vi "test pulse.vi"() -> ()   [LabVIEW 2012]
uses:
  <vilib>/DAQmx/read.llb/DAQmx Read (Digital Bool 1Line 1Point).vi
  <vilib>/DAQmx/create/channels.llb/DAQmx Create Channel (DI-Digital Input).vi
  <vilib>/DAQmx/miscellaneous.llb/DAQmx Fill In Error Info.vi
  <vilib>/express/express arith-compare/Formula/XNode/ExpressFormulaBlockNode.xnode
panel:
  in  "Pi Pulse":bool
  in  "MW post pause":dbl
  in  "Rabi Freq":dbl
  out "Array":dbl[](array[numeric])
  in  "AOM pause + MW delay":dbl
  in  "Sweep range":dbl
  in  "Step size":dbl
  in  "N Loop":i32=25000
  in  "APD signal width":dbl
  out "Run":bool
  in  "AOM Pulse length":dbl=3e-07
  in  "Path to spinapi.dll":path=path "C:/SpinCore/SpinAPI/dll/spinapi64.dll"
  in  "stop":bool
  in  "start/restart":bool
  in  "clock_freq (MHz)":dbl=300.0
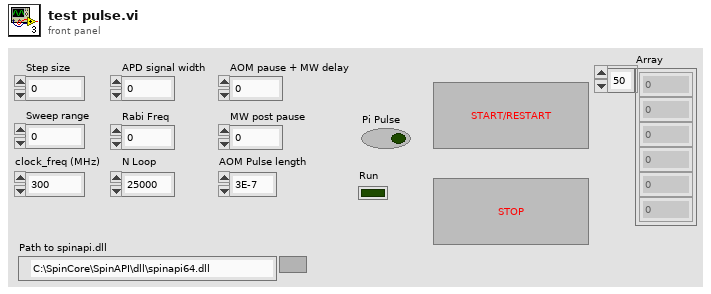
[diagram p1: front panel]
types:
  T1 = cluster{"Instruct Data":i32, "Op Code":i32, "Flags":bool[], "Comments":string, "Time (s)":dbl}[]
  T2 = cluster{"Instruct Data":i32, "Op Code":i32, "Flags":bool[], "Comments":string, "Time (s)":dbl}
  T3 = enum16{"Pulse Program", "Frequency Registers", "TX Phase Registers", "RX Phase Registers"}
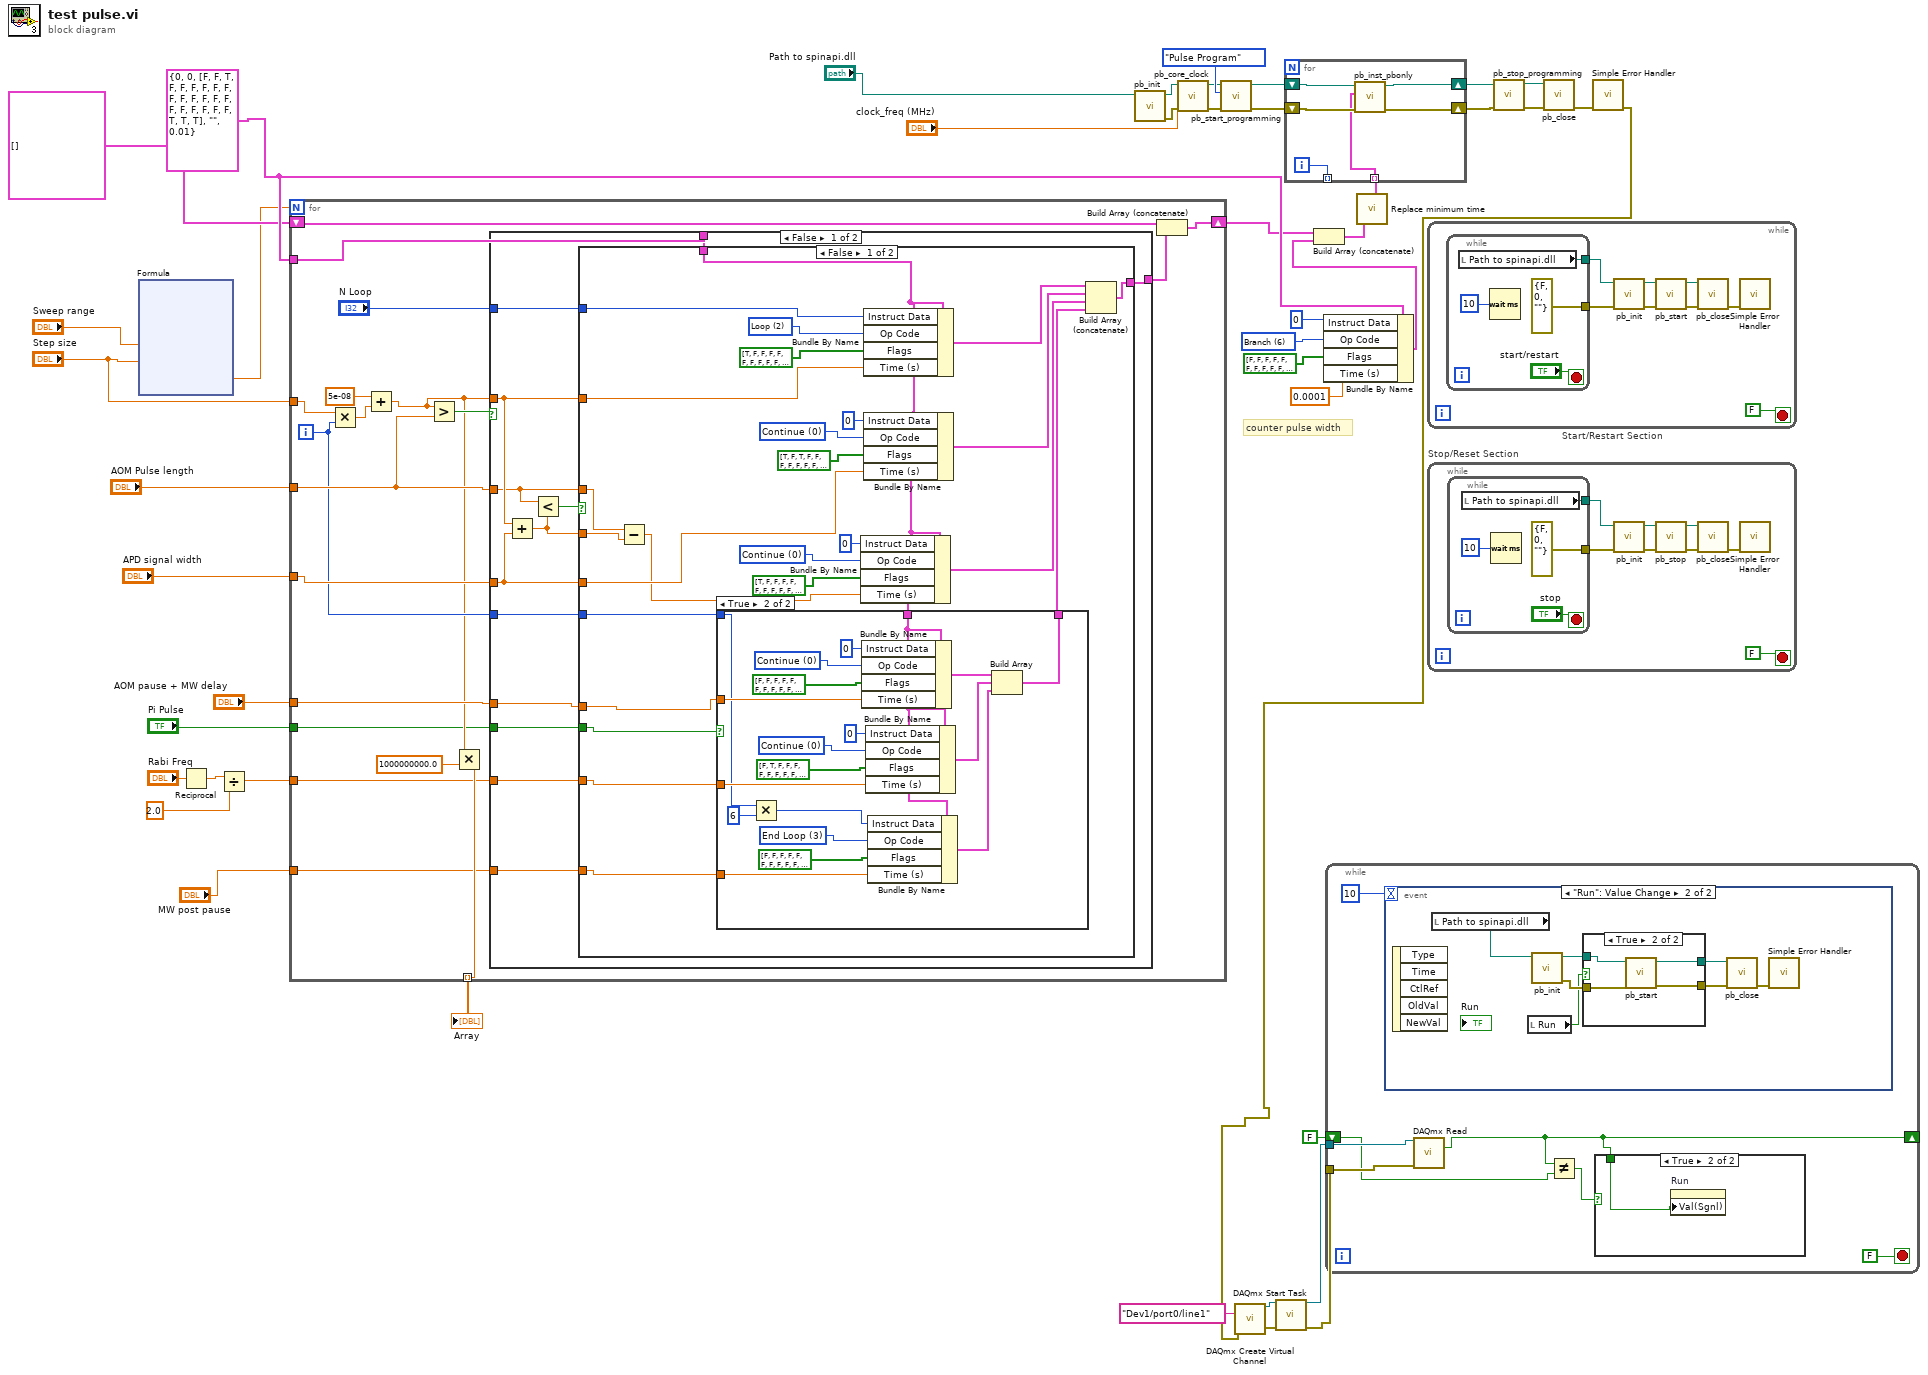
[diagram p0: block diagram]
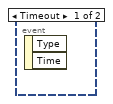
[diagram p2: hidden frame]
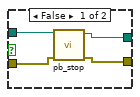
[diagram p3: hidden frame]
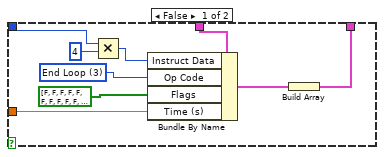
[diagram p5: hidden frame]
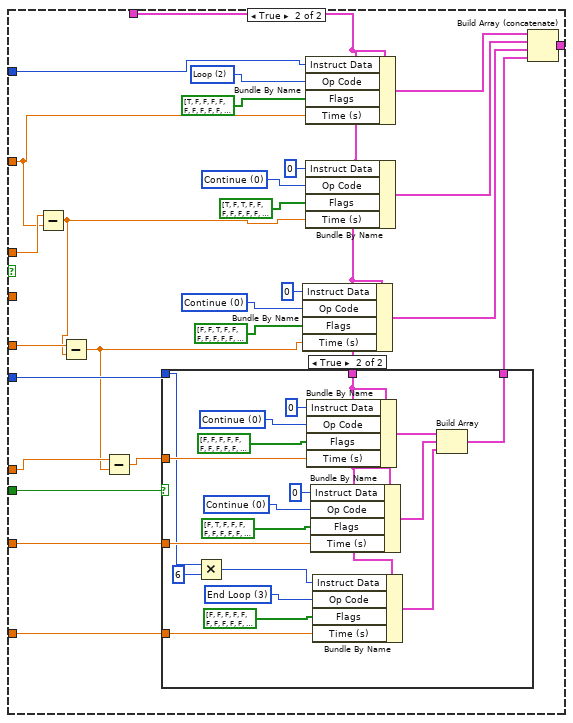
[diagram p6: hidden frame]
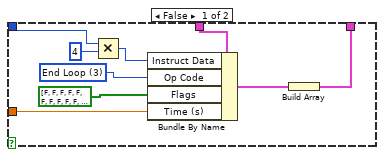
[diagram p7: hidden frame]
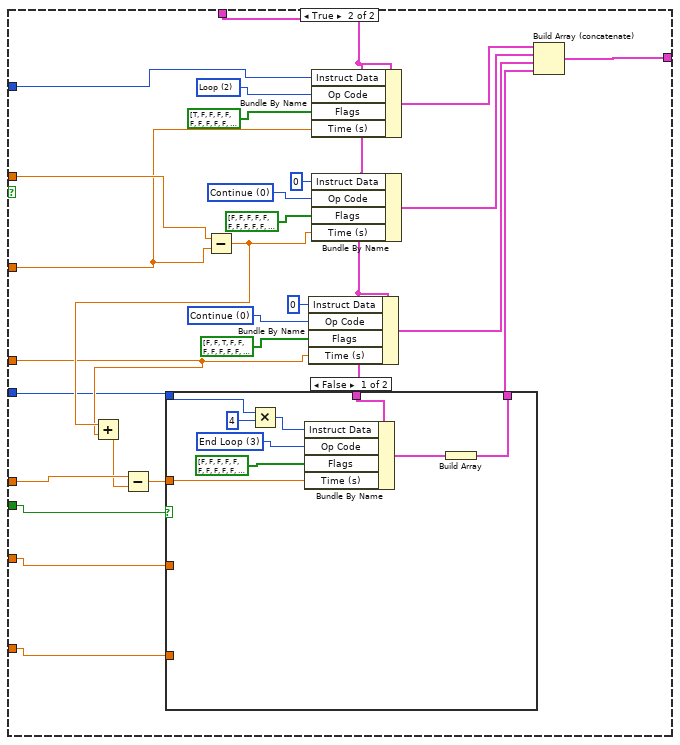
[diagram p8: hidden frame]
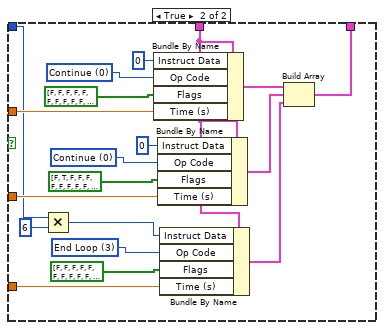
[diagram p9: hidden frame]
diagram:
  w21 = 6 items=["Continue", "Stop", "Loop", "End Loop", "JSR", "RTS", "Branch", "Long Delay", "Wait"] ("Op Code")
  w19 = T2 {"Instruct Data"=0, "Op Code"=0, "Flags"=[FALSE, FALSE, TRUE, FALSE, FALSE, FALSE, FALSE, FALSE, FALSE, FALSE, FALSE, FALSE, FALSE, FALSE, FALSE, FALSE, FALSE, FALSE, FALSE, FALSE, FALSE, TRUE, TRUE, TRUE], "Comments"="", "Time (s)"=0.01} ("PB Inst 2")
  # "counter pulse width"
  n1 = xnode "Formula"("X1"="Sweep range", "X2"="Step size") -> ("Result"=w1:dbl)  [unwired: 1 in, 1 out]
  n2 = Reciprocal(x="Rabi Freq") -> (1/x=w8:dbl)
  n3 = Divide(x=w8, y=2.0) -> (x/y=w7:dbl)
  n4 = for {
    N: w1 -> [_]
    tunnel: w19 -> [w60]
    shift-right: [w62] -> w17
    shift-left: T1 [] -> [w63]
    tunnel: "AOM Pulse length" -> [w54]
    tunnel: "Step size" -> [w58]
    tunnel: "APD signal width" -> [w53]
    tunnel: "AOM pause + MW delay" -> [w51]
    tunnel: [w49] -> w10 mode=indexing
    tunnel: w7 -> [w47]
    tunnel: "MW post pause" -> [w46]
    tunnel: "Pi Pulse" -> [w45]
    i -> [w52]
    n5 = Multiply(x=w58, y=w52) -> (x*y=w57:dbl)
    n6 = Add(x=5e-08, y=w57) -> (x+y=w50:dbl)
    n7 = Greater?(x=w50, y=w54) -> (0:w55:bool)
    n8 = Multiply(x=w50, y=1000000000.0) -> (x*y=w49:dbl)
    n9 = case shown="False" w55 {
      tunnel: [w75 w203] -> w61
      tunnel: w60 -> [w76 w185]
      tunnel: "N Loop" -> [w67 w202]
      tunnel: w54 -> [w72 w195]
      tunnel: w50 -> [w73 w196]
      tunnel: w53 -> [w71 w193]
      tunnel: w52 -> [w70 w190]
      tunnel: w51 -> [w69 w192]
      tunnel: w47 -> [w66 w187]
      tunnel: w46 -> [w65 w186]
      tunnel: w45 -> [w64 w188]
      frame False {
        n10 = Add(x=w73, y=w71) -> (x+y=w68:dbl)
        n11 = Less?(x=w72, y=w68) -> (x < y?=w74:bool)
        n12 = case shown="False" w74 {
          tunnel: w76 -> [w78 w144]
          tunnel: [w90 w142] -> w75
          tunnel: w73 -> [w89 w140]
          tunnel: w72 -> [w87 w141]
          tunnel: w71 -> [w88 w139]
          tunnel: w70 -> [w83 w137]
          tunnel: w69 -> [w82 w136]
          tunnel: w68 -> [w86 _]
          tunnel: w67 -> [w84 w133]
          tunnel: w66 -> [w80 w132]
          tunnel: w65 -> [w79 w131]
          tunnel: w64 -> [w81 w130]
          frame False {
            w99 = 0 items=["Continue", "Stop", "Loop", "End Loop", "JSR", "RTS", "Branch", "Long Delay", "Wait"] ("Op Code")
            w96 = 2 items=["Continue", "Stop", "Loop", "End Loop", "JSR", "RTS", "Branch", "Long Delay", "Wait"] ("Op Code")
            w92 = 0 items=["Continue", "Stop", "Loop", "End Loop", "JSR", "RTS", "Branch", "Long Delay", "Wait"] ("Op Code")
            n13 = Subtract(x=w87, y=w86) -> (x-y=w85:dbl)
            n14 = case shown="True" w81 {
              tunnel: [w102 w111] -> w77
              tunnel: w78 -> [w107 w119]
              tunnel: w83 -> [w106 w117]
              tunnel: w82 -> [w105 w126]
              tunnel: w80 -> [_ w122]
              tunnel: w79 -> [_ w118]
              frame False {
                w104 = 3 items=["Continue", "Stop", "Loop", "End Loop", "JSR", "RTS", "Branch", "Long Delay", "Wait"] ("Op Code")
                n15 = Multiply(x=w106, y=4) -> (x*y=w109:i32)
                n16 = Bundle By Name(cluster=w107, "Instruct Data"=w109, "Op Code"=w104, "Flags"=bool[] [FALSE, FALSE, FALSE, FALSE, FALSE, FALSE, FALSE, FALSE, FALSE, FALSE, FALSE, FALSE, FALSE, FALSE, FALSE, FALSE, FALSE, FALSE, FALSE, FALSE, FALSE, TRUE, TRUE, TRUE], "Time (s)"=w105) -> (w103:T2)
                n17 = Build Array(w103) -> (w102:T1)
              }
              frame True {
                w121 = 3 items=["Continue", "Stop", "Loop", "End Loop", "JSR", "RTS", "Branch", "Long Delay", "Wait"] ("Op Code")
                w125 = 0 items=["Continue", "Stop", "Loop", "End Loop", "JSR", "RTS", "Branch", "Long Delay", "Wait"] ("Op Code")
                w129 = 0 items=["Continue", "Stop", "Loop", "End Loop", "JSR", "RTS", "Branch", "Long Delay", "Wait"] ("Op Code")
                n18 = Multiply(x=w117, y=6) -> (x*y=w115:i32)
                n19 = Bundle By Name(cluster=w119, "Instruct Data"=0, "Op Code"=w129, "Flags"=bool[] [FALSE, FALSE, FALSE, FALSE, FALSE, FALSE, FALSE, FALSE, FALSE, FALSE, FALSE, FALSE, FALSE, FALSE, FALSE, FALSE, FALSE, FALSE, FALSE, FALSE, FALSE, TRUE, TRUE, TRUE], "Time (s)"=w126) -> (w112:T2)
                n20 = Bundle By Name(cluster=w119, "Instruct Data"=0, "Op Code"=w125, "Flags"=bool[] [FALSE, TRUE, FALSE, FALSE, FALSE, FALSE, FALSE, FALSE, FALSE, FALSE, FALSE, FALSE, FALSE, FALSE, FALSE, FALSE, FALSE, FALSE, FALSE, FALSE, FALSE, TRUE, TRUE, TRUE], "Time (s)"=w122) -> (w113:T2)
                n21 = Bundle By Name(cluster=w119, "Instruct Data"=w115, "Op Code"=w121, "Flags"=bool[] [FALSE, FALSE, FALSE, FALSE, FALSE, FALSE, FALSE, FALSE, FALSE, FALSE, FALSE, FALSE, FALSE, FALSE, FALSE, FALSE, FALSE, FALSE, FALSE, FALSE, FALSE, TRUE, TRUE, TRUE], "Time (s)"=w118) -> (w114:T2)
                n22 = Build Array(w112, w113, w114) -> (w111:T1)
              }
            }
            n23 = Bundle By Name(cluster=w78, "Instruct Data"=0, "Op Code"=w92, "Flags"=bool[] [TRUE, FALSE, FALSE, FALSE, FALSE, FALSE, FALSE, FALSE, FALSE, FALSE, FALSE, FALSE, FALSE, FALSE, FALSE, FALSE, FALSE, FALSE, FALSE, FALSE, FALSE, TRUE, TRUE, TRUE], "Time (s)"=w85) -> (w95:T2)
            n24 = Bundle By Name(cluster=w78, "Instruct Data"=w84, "Op Code"=w96, "Flags"=bool[] [TRUE, FALSE, FALSE, FALSE, FALSE, FALSE, FALSE, FALSE, FALSE, FALSE, FALSE, FALSE, FALSE, FALSE, FALSE, FALSE, FALSE, FALSE, FALSE, FALSE, FALSE, TRUE, TRUE, TRUE], "Time (s)"=w89) -> (w101:T2)
            n25 = Bundle By Name(cluster=w78, "Instruct Data"=0, "Op Code"=w99, "Flags"=bool[] [TRUE, FALSE, TRUE, FALSE, FALSE, FALSE, FALSE, FALSE, FALSE, FALSE, FALSE, FALSE, FALSE, FALSE, FALSE, FALSE, FALSE, FALSE, FALSE, FALSE, FALSE, TRUE, TRUE, TRUE], "Time (s)"=w88) -> (w94:T2)
            n26 = Build Array (concatenate)(w101, w94, w95, w77) -> (w90:T1)
          }
          frame True {
            w146 = 0 items=["Continue", "Stop", "Loop", "End Loop", "JSR", "RTS", "Branch", "Long Delay", "Wait"] ("Op Code")
            w149 = 2 items=["Continue", "Stop", "Loop", "End Loop", "JSR", "RTS", "Branch", "Long Delay", "Wait"] ("Op Code")
            w154 = 0 items=["Continue", "Stop", "Loop", "End Loop", "JSR", "RTS", "Branch", "Long Delay", "Wait"] ("Op Code")
            n27 = Subtract(x=w141, y=w140) -> (x-y=w138:dbl)
            n28 = Subtract(x=w139, y=w138) -> (x-y=w135:dbl)
            n29 = Subtract(x=w136, y=w135) -> (x-y=w134:dbl)
            n30 = case shown="True" w130 {
              tunnel: [w156 w165] -> w150
              tunnel: w144 -> [w161 w173]
              tunnel: w137 -> [w160 w171]
              tunnel: w134 -> [w159 w180]
              tunnel: w132 -> [_ w176]
              tunnel: w131 -> [_ w172]
              frame False {
                w158 = 3 items=["Continue", "Stop", "Loop", "End Loop", "JSR", "RTS", "Branch", "Long Delay", "Wait"] ("Op Code")
                n31 = Multiply(x=w160, y=4) -> (x*y=w163:i32)
                n32 = Bundle By Name(cluster=w161, "Instruct Data"=w163, "Op Code"=w158, "Flags"=bool[] [FALSE, FALSE, FALSE, FALSE, FALSE, FALSE, FALSE, FALSE, FALSE, FALSE, FALSE, FALSE, FALSE, FALSE, FALSE, FALSE, FALSE, FALSE, FALSE, FALSE, FALSE, TRUE, TRUE, TRUE], "Time (s)"=w159) -> (w157:T2)
                n33 = Build Array(w157) -> (w156:T1)
              }
              frame True {
                w175 = 3 items=["Continue", "Stop", "Loop", "End Loop", "JSR", "RTS", "Branch", "Long Delay", "Wait"] ("Op Code")
                w179 = 0 items=["Continue", "Stop", "Loop", "End Loop", "JSR", "RTS", "Branch", "Long Delay", "Wait"] ("Op Code")
                w183 = 0 items=["Continue", "Stop", "Loop", "End Loop", "JSR", "RTS", "Branch", "Long Delay", "Wait"] ("Op Code")
                n34 = Multiply(x=w171, y=6) -> (x*y=w169:i32)
                n35 = Bundle By Name(cluster=w173, "Instruct Data"=0, "Op Code"=w183, "Flags"=bool[] [FALSE, FALSE, FALSE, FALSE, FALSE, FALSE, FALSE, FALSE, FALSE, FALSE, FALSE, FALSE, FALSE, FALSE, FALSE, FALSE, FALSE, FALSE, FALSE, FALSE, FALSE, TRUE, TRUE, TRUE], "Time (s)"=w180) -> (w166:T2)
                n36 = Bundle By Name(cluster=w173, "Instruct Data"=0, "Op Code"=w179, "Flags"=bool[] [FALSE, TRUE, FALSE, FALSE, FALSE, FALSE, FALSE, FALSE, FALSE, FALSE, FALSE, FALSE, FALSE, FALSE, FALSE, FALSE, FALSE, FALSE, FALSE, FALSE, FALSE, TRUE, TRUE, TRUE], "Time (s)"=w176) -> (w167:T2)
                n37 = Bundle By Name(cluster=w173, "Instruct Data"=w169, "Op Code"=w175, "Flags"=bool[] [FALSE, FALSE, FALSE, FALSE, FALSE, FALSE, FALSE, FALSE, FALSE, FALSE, FALSE, FALSE, FALSE, FALSE, FALSE, FALSE, FALSE, FALSE, FALSE, FALSE, FALSE, TRUE, TRUE, TRUE], "Time (s)"=w172) -> (w168:T2)
                n38 = Build Array(w166, w167, w168) -> (w165:T1)
              }
            }
            n39 = Bundle By Name(cluster=w144, "Instruct Data"=0, "Op Code"=w154, "Flags"=bool[] [FALSE, FALSE, TRUE, FALSE, FALSE, FALSE, FALSE, FALSE, FALSE, FALSE, FALSE, FALSE, FALSE, FALSE, FALSE, FALSE, FALSE, FALSE, FALSE, FALSE, FALSE, TRUE, TRUE, TRUE], "Time (s)"=w135) -> (w151:T2)
            n40 = Bundle By Name(cluster=w144, "Instruct Data"=w133, "Op Code"=w149, "Flags"=bool[] [TRUE, FALSE, FALSE, FALSE, FALSE, FALSE, FALSE, FALSE, FALSE, FALSE, FALSE, FALSE, FALSE, FALSE, FALSE, FALSE, FALSE, FALSE, FALSE, FALSE, FALSE, TRUE, TRUE, TRUE], "Time (s)"=w140) -> (w143:T2)
            n41 = Bundle By Name(cluster=w144, "Instruct Data"=0, "Op Code"=w146, "Flags"=bool[] [TRUE, FALSE, TRUE, FALSE, FALSE, FALSE, FALSE, FALSE, FALSE, FALSE, FALSE, FALSE, FALSE, FALSE, FALSE, FALSE, FALSE, FALSE, FALSE, FALSE, FALSE, TRUE, TRUE, TRUE], "Time (s)"=w138) -> (w152:T2)
            n42 = Build Array (concatenate)(w143, w152, w151, w150) -> (w142:T1)
          }
        }
      }
      frame True {
        w198 = 0 items=["Continue", "Stop", "Loop", "End Loop", "JSR", "RTS", "Branch", "Long Delay", "Wait"] ("Op Code")
        w201 = 2 items=["Continue", "Stop", "Loop", "End Loop", "JSR", "RTS", "Branch", "Long Delay", "Wait"] ("Op Code")
        w208 = 0 items=["Continue", "Stop", "Loop", "End Loop", "JSR", "RTS", "Branch", "Long Delay", "Wait"] ("Op Code")
        n43 = Subtract(x=w196, y=w195) -> (x-y=w194:dbl)
        n44 = Add(x=w194, y=w193) -> (x+y=w191:dbl)
        n45 = Subtract(x=w192, y=w191) -> (x-y=w189:dbl)
        n46 = case shown="False" w188 {
          tunnel: [w210 w219] -> w184
          tunnel: w185 -> [w215 w227]
          tunnel: w190 -> [w214 w225]
          tunnel: w189 -> [w213 w234]
          tunnel: w187 -> [_ w230]
          tunnel: w186 -> [_ w226]
          frame False {
            w212 = 3 items=["Continue", "Stop", "Loop", "End Loop", "JSR", "RTS", "Branch", "Long Delay", "Wait"] ("Op Code")
            n47 = Multiply(x=w214, y=4) -> (x*y=w217:i32)
            n48 = Bundle By Name(cluster=w215, "Instruct Data"=w217, "Op Code"=w212, "Flags"=bool[] [FALSE, FALSE, FALSE, FALSE, FALSE, FALSE, FALSE, FALSE, FALSE, FALSE, FALSE, FALSE, FALSE, FALSE, FALSE, FALSE, FALSE, FALSE, FALSE, FALSE, FALSE, TRUE, TRUE, TRUE], "Time (s)"=w213) -> (w211:T2)
            n49 = Build Array(w211) -> (w210:T1)
          }
          frame True {
            w229 = 3 items=["Continue", "Stop", "Loop", "End Loop", "JSR", "RTS", "Branch", "Long Delay", "Wait"] ("Op Code")
            w233 = 0 items=["Continue", "Stop", "Loop", "End Loop", "JSR", "RTS", "Branch", "Long Delay", "Wait"] ("Op Code")
            w237 = 0 items=["Continue", "Stop", "Loop", "End Loop", "JSR", "RTS", "Branch", "Long Delay", "Wait"] ("Op Code")
            n50 = Multiply(x=w225, y=6) -> (x*y=w223:i32)
            n51 = Bundle By Name(cluster=w227, "Instruct Data"=0, "Op Code"=w237, "Flags"=bool[] [FALSE, FALSE, FALSE, FALSE, FALSE, FALSE, FALSE, FALSE, FALSE, FALSE, FALSE, FALSE, FALSE, FALSE, FALSE, FALSE, FALSE, FALSE, FALSE, FALSE, FALSE, TRUE, TRUE, TRUE], "Time (s)"=w234) -> (w220:T2)
            n52 = Bundle By Name(cluster=w227, "Instruct Data"=0, "Op Code"=w233, "Flags"=bool[] [FALSE, TRUE, FALSE, FALSE, FALSE, FALSE, FALSE, FALSE, FALSE, FALSE, FALSE, FALSE, FALSE, FALSE, FALSE, FALSE, FALSE, FALSE, FALSE, FALSE, FALSE, TRUE, TRUE, TRUE], "Time (s)"=w230) -> (w221:T2)
            n53 = Bundle By Name(cluster=w227, "Instruct Data"=w223, "Op Code"=w229, "Flags"=bool[] [FALSE, FALSE, FALSE, FALSE, FALSE, FALSE, FALSE, FALSE, FALSE, FALSE, FALSE, FALSE, FALSE, FALSE, FALSE, FALSE, FALSE, FALSE, FALSE, FALSE, FALSE, TRUE, TRUE, TRUE], "Time (s)"=w226) -> (w222:T2)
            n54 = Build Array(w220, w221, w222) -> (w219:T1)
          }
        }
        n55 = Bundle By Name(cluster=w185, "Instruct Data"=0, "Op Code"=w208, "Flags"=bool[] [FALSE, FALSE, TRUE, FALSE, FALSE, FALSE, FALSE, FALSE, FALSE, FALSE, FALSE, FALSE, FALSE, FALSE, FALSE, FALSE, FALSE, FALSE, FALSE, FALSE, FALSE, TRUE, TRUE, TRUE], "Time (s)"=w193) -> (w204:T2)
        n56 = Bundle By Name(cluster=w185, "Instruct Data"=w202, "Op Code"=w201, "Flags"=bool[] [TRUE, FALSE, FALSE, FALSE, FALSE, FALSE, FALSE, FALSE, FALSE, FALSE, FALSE, FALSE, FALSE, FALSE, FALSE, FALSE, FALSE, FALSE, FALSE, FALSE, FALSE, TRUE, TRUE, TRUE], "Time (s)"=w195) -> (w206:T2)
        n57 = Bundle By Name(cluster=w185, "Instruct Data"=0, "Op Code"=w198, "Flags"=bool[] [FALSE, FALSE, FALSE, FALSE, FALSE, FALSE, FALSE, FALSE, FALSE, FALSE, FALSE, FALSE, FALSE, FALSE, FALSE, FALSE, FALSE, FALSE, FALSE, FALSE, FALSE, TRUE, TRUE, TRUE], "Time (s)"=w194) -> (w205:T2)
        n58 = Build Array (concatenate)(w206, w205, w204, w184) -> (w203:T1)
      }
    }
    n59 = Build Array (concatenate)(w63, w61) -> (w62:T1)
  }
  "Array" <- w10
  n60 = call "pb_init.vi"("path in"="Path to spinapi.dll") -> ("error out"=w39:errorcluster, "path out"=w41:path)  [unwired: 3 in, 6 out]
  n61 = call "pb_core_clock.vi"("error in (no error)"=w39, "clock_freq (MHz)"="clock_freq (MHz)", "path in"=w41) -> ("error out"=w38:errorcluster, "path out"=w40:path)  [unwired: 7 in]
  n62 = call "pb_start_programming.vi"("error in (no error)"=w38, "Device"=T3."Pulse Program", "path in"=w40) -> ("error out"=w35:errorcluster, "path out"=w36:path)  [unwired: 1 in, 6 out]
  n63 = Bundle By Name(cluster=w19, "Instruct Data"=0, "Op Code"=w21, "Flags"=bool[] [FALSE, FALSE, FALSE, FALSE, FALSE, FALSE, FALSE, FALSE, FALSE, FALSE, FALSE, FALSE, FALSE, FALSE, FALSE, FALSE, FALSE, FALSE, FALSE, FALSE, FALSE, TRUE, TRUE, TRUE], "Time (s)"=0.0001) -> (w18:T2)
  n64 = Build Array (concatenate)(w17, w18) -> (w3:T1)
  n65 = call "Replace minimum time.vi"("Array"=w3) -> ("Array 2"=w2:T1)  [unwired: 10 in]
  n66 = for {
    shift-right: [w241] -> w34
    shift-left: w36 -> [w243]
    shift-right: [w240] -> w33
    shift-left: w35 -> [w242]
    tunnel: [w239] -> _ mode=indexing
    tunnel: w2 -> [w238] mode=indexing
    i -> [w239]
    n67 = call "pb_inst_pbonly.vi"("error in (no error)"=w242, "PB Instruction"=w238, "path in"=w243) -> ("error out"=w240:errorcluster, "path out"=w241:path)  [unwired: 2 in, 5 out]
  }
  n68 = while "Start/Restart Section" {
    stop <- FALSE stop-if-true
    n69 = while {
      tunnel: [errorcluster {"status"=FALSE, "code"=0, "source"=""} ("error in (no error)")] -> w248
      tunnel: [w252] -> w244
      stop <- "start/restart" stop-if-true
      n70 = local read "Path to spinapi.dll"() -> (w252:path)
      n71 = Wait (ms)(milliseconds to wait=u32 10) -> ()  [unwired: 1 out]
    }
    n72 = call "pb_init.vi"("error in (no error)"=w248, "path in"=w244) -> ("error out"=w247:errorcluster, "path out"=w250:path)  [unwired: 1 in, 7 out]
    n73 = call "pb_start.vi"("error in (no error)"=w247, "path in"=w250) -> ("error out"=w246:errorcluster, "path out"=w251:path)  [unwired: 1 in, 7 out]
    n74 = call "pb_close.vi"("error in (no error)"=w246, "path in"=w251) -> ("error out"=w245:errorcluster)  [unwired: 9 out]
    n75 = call <vilib>:"Simple Error Handler.vi"("error in (no error)"=w245) -> ()  [unwired: 1 in, 8 out]
  }
  n76 = while "Stop/Reset Section" {
    stop <- FALSE stop-if-true
    n77 = while {
      tunnel: [errorcluster {"status"=FALSE, "code"=0, "source"=""} ("error in (no error)")] -> w260
      tunnel: [w264] -> w256
      stop <- "stop" stop-if-true
      n78 = local read "Path to spinapi.dll"() -> (w264:path)
      n79 = Wait (ms)(milliseconds to wait=u32 10) -> ()  [unwired: 1 out]
    }
    n80 = call "pb_init.vi"("error in (no error)"=w260, "path in"=w256) -> ("error out"=w259:errorcluster, "path out"=w262:path)  [unwired: 1 in, 7 out]
    n81 = call "pb_stop.vi"("error in (no error)"=w259, "path in"=w262) -> ("error out"=w258:errorcluster, "path out"=w263:path)  [unwired: 8 out]
    n82 = call "pb_close.vi"("error in (no error)"=w258, "path in"=w263) -> ("error out"=w257:errorcluster)  [unwired: 9 out]
    n83 = call <vilib>:"Simple Error Handler.vi"("error in (no error)"=w257) -> ()  [unwired: 1 in, 8 out]
  }
  n84 = call "pb_stop_programming.vi"("error in (no error)"=w33, "path in"=w34) -> ("error out"=w42:errorcluster, "path out"=w43:path)  [unwired: 1 in, 7 out]
  n85 = call "pb_close.vi"("error in (no error)"=w42, "path in"=w43) -> ("error out"=w31:errorcluster)  [unwired: 9 out]
  n86 = call <vilib>:"Simple Error Handler.vi"("error in (no error)"=w31) -> ("error out"=w27:errorcluster)  [unwired: 1 in, 7 out]
  n87 = call-poly <vilib>:"DAQmx Create Virtual Channel.vi"("lines"=tag "Dev1/port0/line1", "error in"=w27) -> ("task out"=w25:refnum<k21>, "error out"=w24:errorcluster)  [unwired: 12 in]
  n88 = call <vilib>:"DAQmx Start Task.vi"("task/channels in"=w25, "error in"=w24) -> ("task out"=w26:refnum<k21>, "error out"=w29:errorcluster)  [unwired: 12 in]
  n89 = while {
    tunnel: w26 -> [w274]
    tunnel: w29 -> [w273]
    shift-right: [w270] -> _
    shift-left: FALSE ("data") -> [w272]
    stop <- FALSE stop-if-true
    n90 = event shown="[1] \"Run\": Value Change" {
      selector: _ -> [_ _]
      dyn-events: _ -> [_ _]
      timeout: 10 -> [_ _]
      event Timeout {
        n91 = event-data() -> ()  [unwired: 1 in, 2 out]
      }
      event "Run": Value Change {
        n92 = event-data() -> ()  [unwired: 1 in, 5 out]
        n93 = local read "Path to spinapi.dll"() -> (w275:path)
        n94 = local read "Run"() -> (w279:bool)
        n95 = call "pb_init.vi"("path in"=w275) -> ("error out"=w280:errorcluster, "path out"=w281:path)  [unwired: 2 in, 7 out]
        n96 = case shown="True" w279 {
          tunnel: w281 -> [w285 w289]
          tunnel: w280 -> [w284 w288]
          tunnel: [w283 w287] -> w277
          tunnel: [w282 w286] -> w276
          frame False {
            n97 = call "pb_stop.vi"("error in (no error)"=w284, "path in"=w285) -> ("error out"=w282:errorcluster, "path out"=w283:path)  [unwired: 8 out]
          }
          frame True {
            n98 = call "pb_start.vi"("error in (no error)"=w288, "path in"=w289) -> ("error out"=w286:errorcluster, "path out"=w287:path)  [unwired: 1 in, 7 out]
          }
        }
        n99 = call "pb_close.vi"("error in (no error)"=w276, "path in"=w277) -> ("error out"=w278:errorcluster)  [unwired: 9 out]
        n100 = call <vilib>:"Simple Error Handler.vi"("error in (no error)"=w278) -> ()  [unwired: 1 in, 8 out]
      }
    }
    n101 = call-poly <vilib>:"DAQmx Read.vi"("task/channels in"=w274, "error in"=w273) -> ("data"=w270:bool)  [unwired: 11 in, 2 out]
    n102 = Not Equal?(x=w270, y=w272) -> (x != y?=w271:bool)
    n103 = case shown="True" w271 {
      tunnel: w270 -> [_ w290]
      frame False {
      }
      frame True {
        n104 = property on="Run" class="Bool (strict)"("Val(Sgnl)"=w290) -> ()  [unwired: 2 in, 2 out]
      }
    }
  }
